vi "ORS_window.vi"(6 "window parameter":dbl=nan, 8 "window":T1=62 items=["Rectangle"=0, "Hanning"=1, "Hamming"=2, "Blackman-Harris"=3, "Exact Blackman"=4, "Blackman"=5, "Flat Top"=6, "4 Term B-Harris "=7, "7 Term B-Harris"=8, "Low Sidelobe"=9, "Blackman Nuttall"=11, "Triangle"=30, "Bartlett-Hanning"=31, "Bohman"=32, "Parzen"=33, "Welch"=34, "Kaiser"=60, "Dolph-Chebyshev"=61, "Gaussian"=62], 9 "Window size":i32) -> (0 "Shape factor/window":dbl[](graph))   [LabVIEW 2014]
uses:
  <vilib>/Analysis/4window.llb/windowTd.ctl
  <vilib>/Analysis/4window.llb/Symmetric Window (DBL).vi
  <vilib>/Analysis/NI_AALPro.lvlib
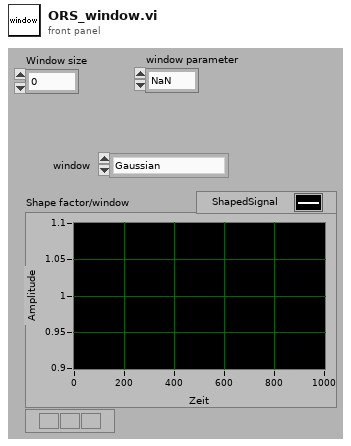
[diagram p1: front panel]
types:
  T1 = typedef "NI_AALPro.lvlib/windowTd.ctl" = u32
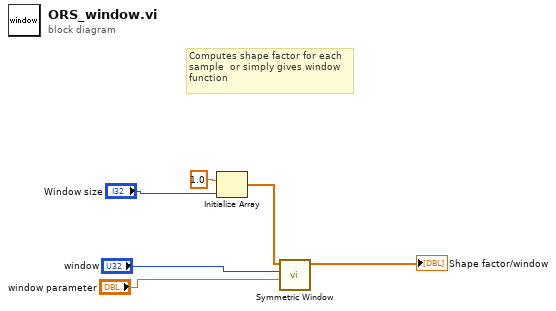
[diagram p0: block diagram]
diagram:
  # "Computes shape factor for each sample  or simply gives window function"
  n1 = Initialize Array(1.0 ("element"), "Window size") -> (w1:dbl[])
  n2 = call-poly <vilib>:"Symmetric Window.vi"("window parameter"="window parameter", "window"="window", "X"=w1) -> ("Windowed X"=→"Shape factor/window":dbl[])  [unwired: 7 in, 1 out]
